vi "ExternalIO.vi"(0 "Element Set":string) -> ()   [LabVIEW 2011]
uses:
  SesWrapper/SesWrapper.lvlib
panel:
  in  "Instrument Configuration File":string
  in  "Working Directory":string
  out "Ports Out":string[](array[string])
  out "External IO":dbl[][](graph)
  in  "Use Detector":u8
  in  "Use External IO":u8
  in  "Stop":bool
  in  "Accumulate":bool
  in  "Detector Region":T1={"firstXChannel_"=1, "lastXChannel_"=1392, "firstYChannel_"=1, "lastYChannel_"=519, "slices_"=519, "adcMode_"=1}
  in  "Region":T2={"fixed_"=0, "highEnergy_"=500.0, "lowEnergy_"=0.0, "centerEnergy_"=0.0, "energyStep_"=10.0, "dwellTime_"=80}
  in  "Pass Energy":dbl=150.0
  in  "Lens Mode":string="Transmission"
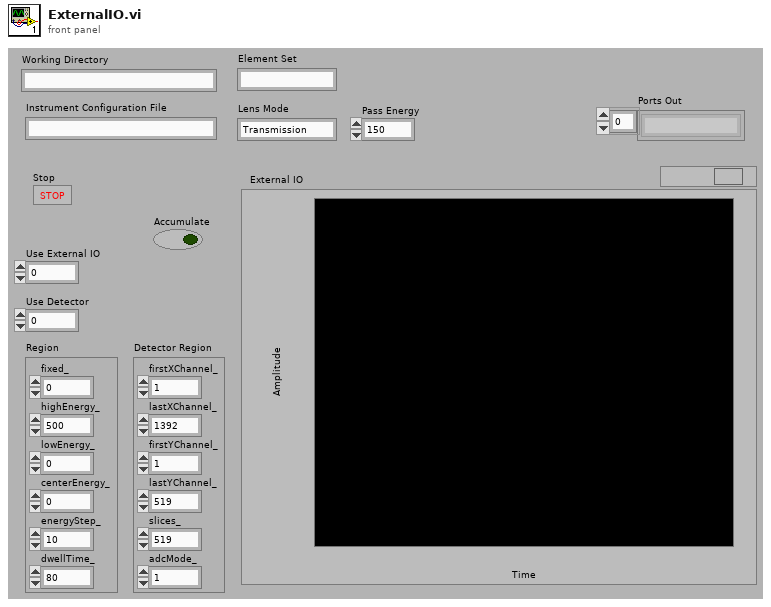
[diagram p1: front panel]
types:
  T1 = cluster{"firstXChannel_":i32, "lastXChannel_":i32, "firstYChannel_":i32, "lastYChannel_":i32, "slices_":i32, "adcMode_":u8}
  T2 = cluster{"fixed_":u8, "highEnergy_":dbl, "lowEnergy_":dbl, "centerEnergy_":dbl, "energyStep_":dbl, "dwellTime_":i32}
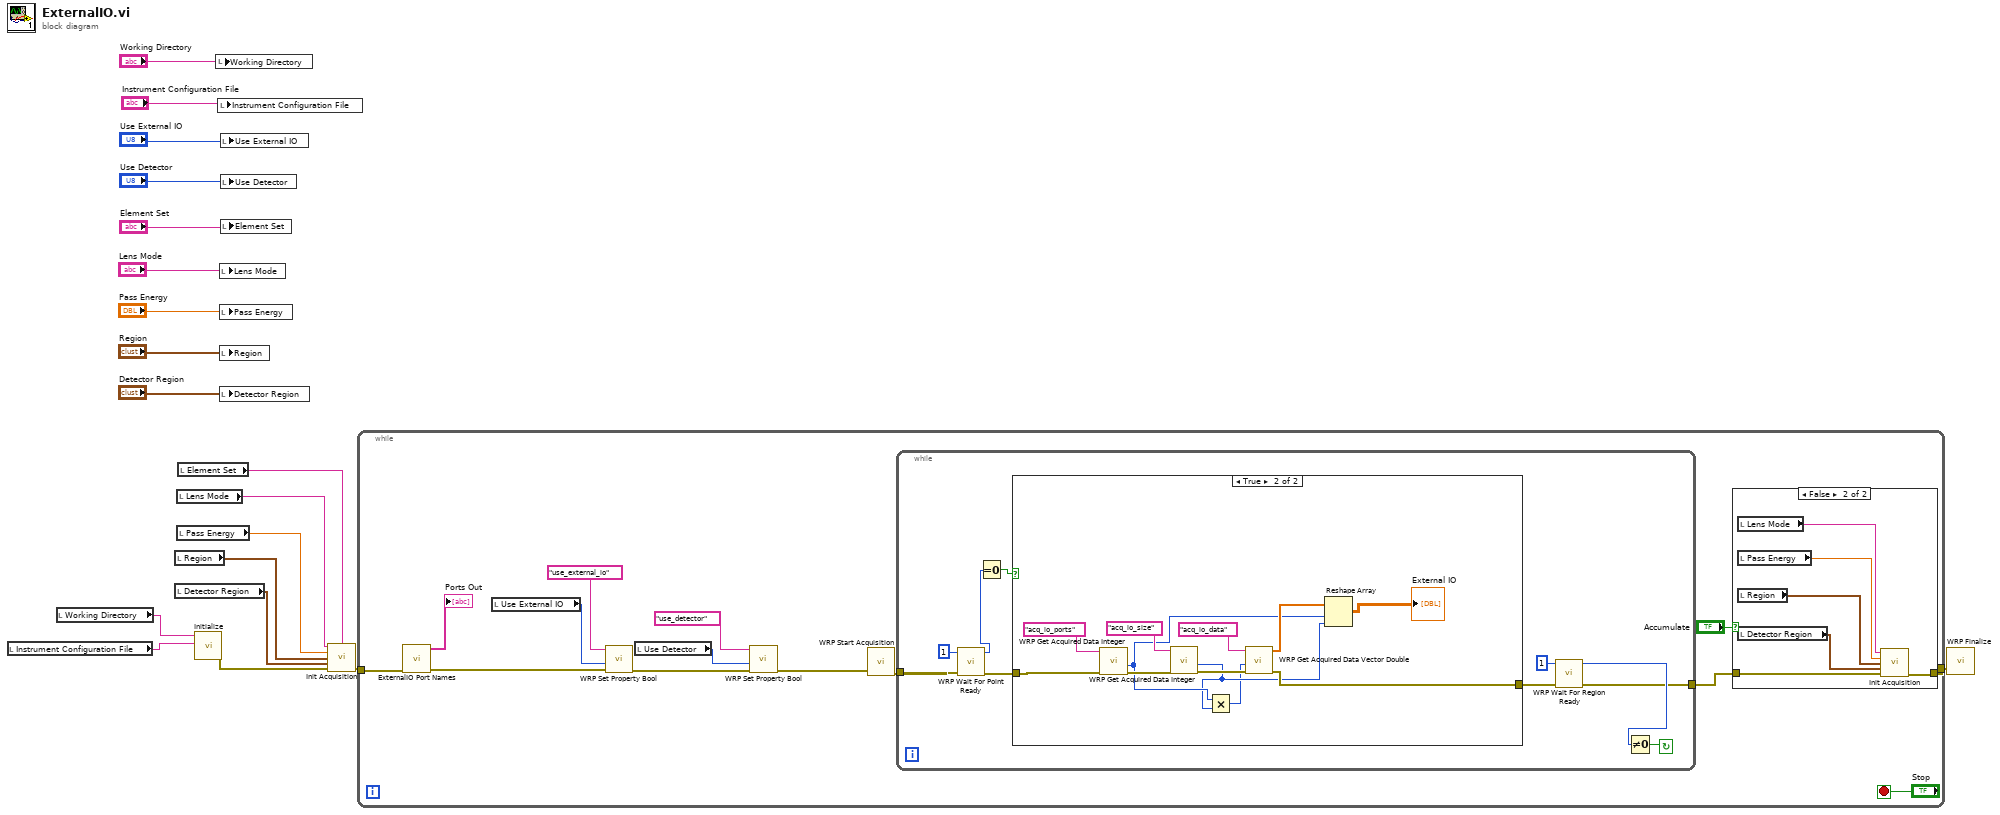
[diagram p0: block diagram]
diagram:
  n1 = local read "Instrument Configuration File"() -> (w1:string)
  n2 = local read "Working Directory"() -> (w2:string)
  n3 = local read "Region"() -> (w13:T2)
  n4 = local read "Detector Region"() -> (w12:T1)
  n5 = local read "Lens Mode"() -> (w11:string)
  n6 = local read "Pass Energy"() -> (w14:dbl)
  n7 = local read "Element Set"() -> (w5:string)
  n8 = call "Initialize.vi"("Instrument Configuration File"=w1, "working_directory"=w2) -> ("error out"=w15:errorcluster)  [unwired: 9 in]
  n9 = local write "Working Directory"("Working Directory") -> ()
  n10 = local write "Instrument Configuration File"("Instrument Configuration File") -> ()
  n11 = local write "Lens Mode"("Lens Mode") -> ()
  n12 = local write "Pass Energy"("Pass Energy") -> ()
  n13 = local write "Region"("Region") -> ()
  n14 = local write "Detector Region"("Detector Region") -> ()
  n15 = local write "Use External IO"("Use External IO") -> ()
  n16 = local write "Use Detector"("Use Detector") -> ()
  n17 = local write "Element Set"("Element Set") -> ()
  n18 = call "Init Acquisition.vi"("Lens Mode"=w11, "element_set"=w5, "Pass Energy"=w14, "Region"=w13, "Detector Region"=w12, "error in (no error)"=w15) -> ("error out"=w9:errorcluster)  [unwired: 4 in, 5 out]
  n19 = while {
    tunnel: [w30] -> w10
    tunnel: w9 -> [w24]
    stop <- "Stop" stop-if-true
    n20 = call "ExternalIO Port Names.vi"("error in (no error)"=w24) -> ("error out"=w23:errorcluster, "Ports Out"=→"Ports Out":string[])  [unwired: 9 in]
    n21 = local read "Use External IO"() -> (w21:u8)
    n22 = call "WRP Set Property Bool.vi"("error in (no error)"=w23, "value"=w21, "property"="use_external_io") -> ("error out"=w27:errorcluster)  [unwired: 7 in, 1 out]
    n23 = local read "Use Detector"() -> (w20:u8)
    n24 = call "WRP Set Property Bool.vi"("error in (no error)"=w27, "value"=w20, "property"="use_detector") -> ("error out"=w26:errorcluster)  [unwired: 7 in, 1 out]
    n25 = call "WRP Start Acquisition.vi"("error in (no error)"=w26) -> ("error out"=w33:errorcluster)  [unwired: 9 in, 1 out]
    n26 = while {
      tunnel: w33 -> [w49]
      tunnel: [w41] -> w29
      stop <- w50 continue-if-true
      n27 = call "WRP Wait For Point Ready.vi"("error in (no error)"=w49, "timeout_ms"=1) -> ("error out"=w47:errorcluster, "function return"=w42:i32)  [unwired: 8 in]
      n28 = Equal To 0?(x=w42) -> (x = 0?=w43:bool)
      n29 = case shown="True" w43 {
        tunnel: w47 -> [w51 w62]
        tunnel: [w51 w55] -> w46
        frame False {
        }
        frame True {
          n30 = call "WRP Get Acquired Data Integer.vi"("error in (no error)"=w62, "parameter"="acq_io_ports") -> ("error out"=w60:errorcluster, "size out"=w54:i32)  [unwired: 6 in, 2 out]
          n31 = call "WRP Get Acquired Data Integer.vi"("error in (no error)"=w60, "parameter"="acq_io_size") -> ("error out"=w59:errorcluster, "size out"=w53:i32)  [unwired: 6 in, 2 out]
          n32 = Multiply(x=w54, y=w53) -> (x*y=w52:i32)
          n33 = call "WRP Get Acquired Data Vector Double.vi"("error in (no error)"=w59, "size"=w52, "parameter"="acq_io_data") -> ("error out"=w55:errorcluster, "data"=w57:dbl[])  [unwired: 5 in, 2 out]
          n34 = Reshape Array(w57, w54, w53) -> (→"External IO":dbl[][])
        }
      }
      n35 = call "WRP Wait For Region Ready.vi"("error in (no error)"=w46, "timeout_ms"=1) -> ("error out"=w41:errorcluster, "function return"=w45:i32)  [unwired: 8 in]
      n36 = Not Equal To 0?(x=w45) -> (x != 0?=w50:bool)
    }
    n37 = case shown="False" "Accumulate" {
      tunnel: [w34 w40] -> w30
      tunnel: w29 -> [w34 w39]
      frame True {
      }
      frame False {
        n38 = local read "Lens Mode"() -> (w38:string)
        n39 = local read "Pass Energy"() -> (w37:dbl)
        n40 = local read "Region"() -> (w36:T2)
        n41 = local read "Detector Region"() -> (w35:T1)
        n42 = call "Init Acquisition.vi"("Lens Mode"=w38, "Pass Energy"=w37, "Region"=w36, "Detector Region"=w35, "error in (no error)"=w39) -> ("error out"=w40:errorcluster)  [unwired: 5 in, 5 out]
      }
    }
  }
  n43 = call "WRP Finalize.vi"("error in (no error)"=w10) -> ()  [unwired: 9 in, 2 out]
